vi "LRF offset.vi"(3 "Robot position":dbl[](array[numeric]), 4 "Robot direction":dbl(slide) scale=3.2..-3.2, 5 "LRF offset":dbl) -> (0 "Dy":dbl, 1 "Dx":dbl, 2 "LRF position":dbl[](array[numeric]))   [LabVIEW 2009]
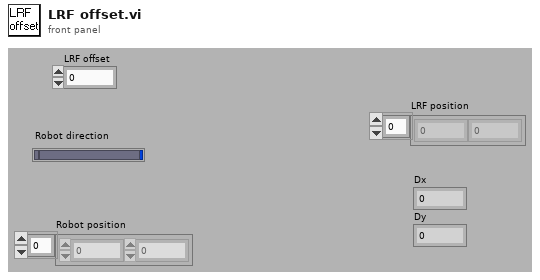
[diagram p1: front panel]
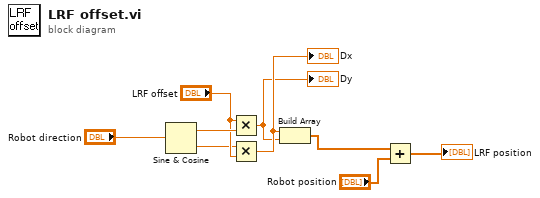
[diagram p0: block diagram]
diagram:
  n1 = Sine & Cosine(0:"Robot direction") -> (1:w8:dbl, 2:w6:dbl)
  n2 = Multiply(x="LRF offset", y=w8) -> (x*y=w4:dbl)
  "Dy" <- w4
  n3 = Multiply(x=w6, y="LRF offset") -> (x*y=w5:dbl)
  "Dx" <- w5
  n4 = Build Array(w5, w4) -> (w3:dbl[])
  n5 = Add(x=w3, y="Robot position") -> (x+y=→"LRF position":dbl[])
